vi "ArrayAdd.vi"(0 "InputArray1":dbl[](array[numeric]), 11 "InputArray2":dbl[](array[numeric])) -> (15 "OutputArray":dbl[](array[numeric]))   [LabVIEW 2016]
panel:
  # "Adds the two input arrays together\n\nIf Array2 is empty, returns Array1 to preserve\narray sizes."
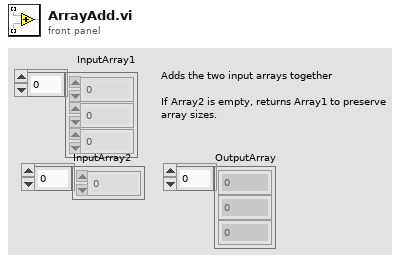
[diagram p1: front panel]
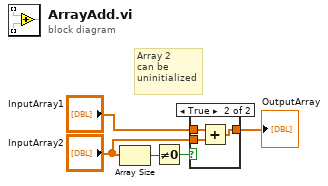
[diagram p0: block diagram]
diagram:
  # "Array 2\ncan be\nuninitialized"
  n1 = Array Size(array="InputArray2") -> (size(s)=w1:i32)
  n2 = Not Equal To 0?(x=w1) -> (x != 0?=w2:bool)
  n3 = case shown="True" w2 {
    tunnel: "InputArray1" -> [w6 w9]
    tunnel: "InputArray2" -> [_ w8]
    tunnel: [w6 w7] -> w4
    frame False {
    }
    frame True {
      n4 = Add(x=w9, y=w8) -> (x+y=w7:dbl[])
    }
  }
  "OutputArray" <- w4
